vi "Demo.vi"() -> ()   [LabVIEW 2012]
panel:
  in  "MVOCX":refnum<k7>(container)
  out "采集BMP图像":picture
  in  "?":bool
  out "采集JPG图像":picture
  in  "Stop":bool
  in  "?":bool
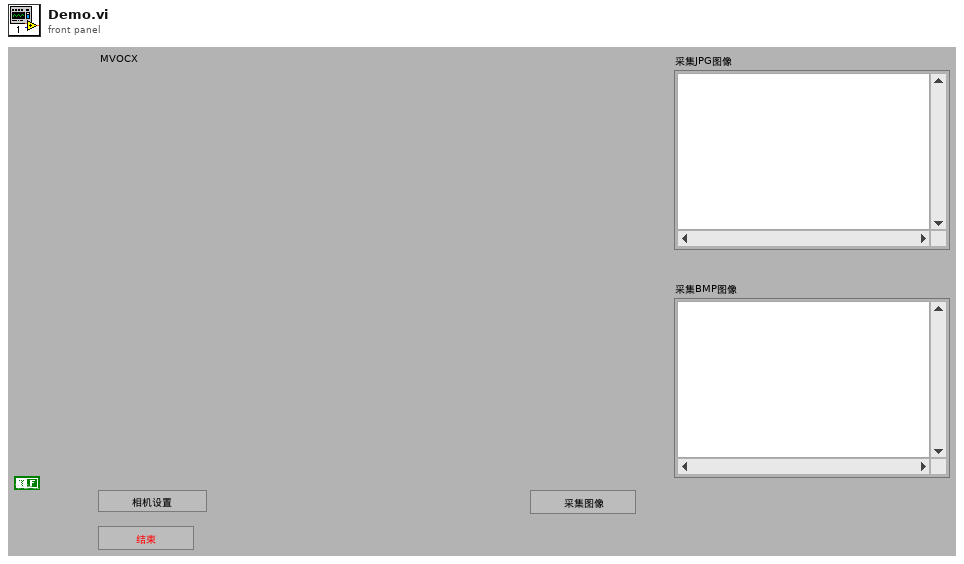
[diagram p1: front panel]
types:
  T1 = typedef "imagedata.ctl" = cluster{"image type":i32, "image depth":i32, "image":u8[], "mask":u8[], "colors":u32[], "Rectangle":cluster{"left":i16, "top":i16, "right":i16, "bottom":i16}}
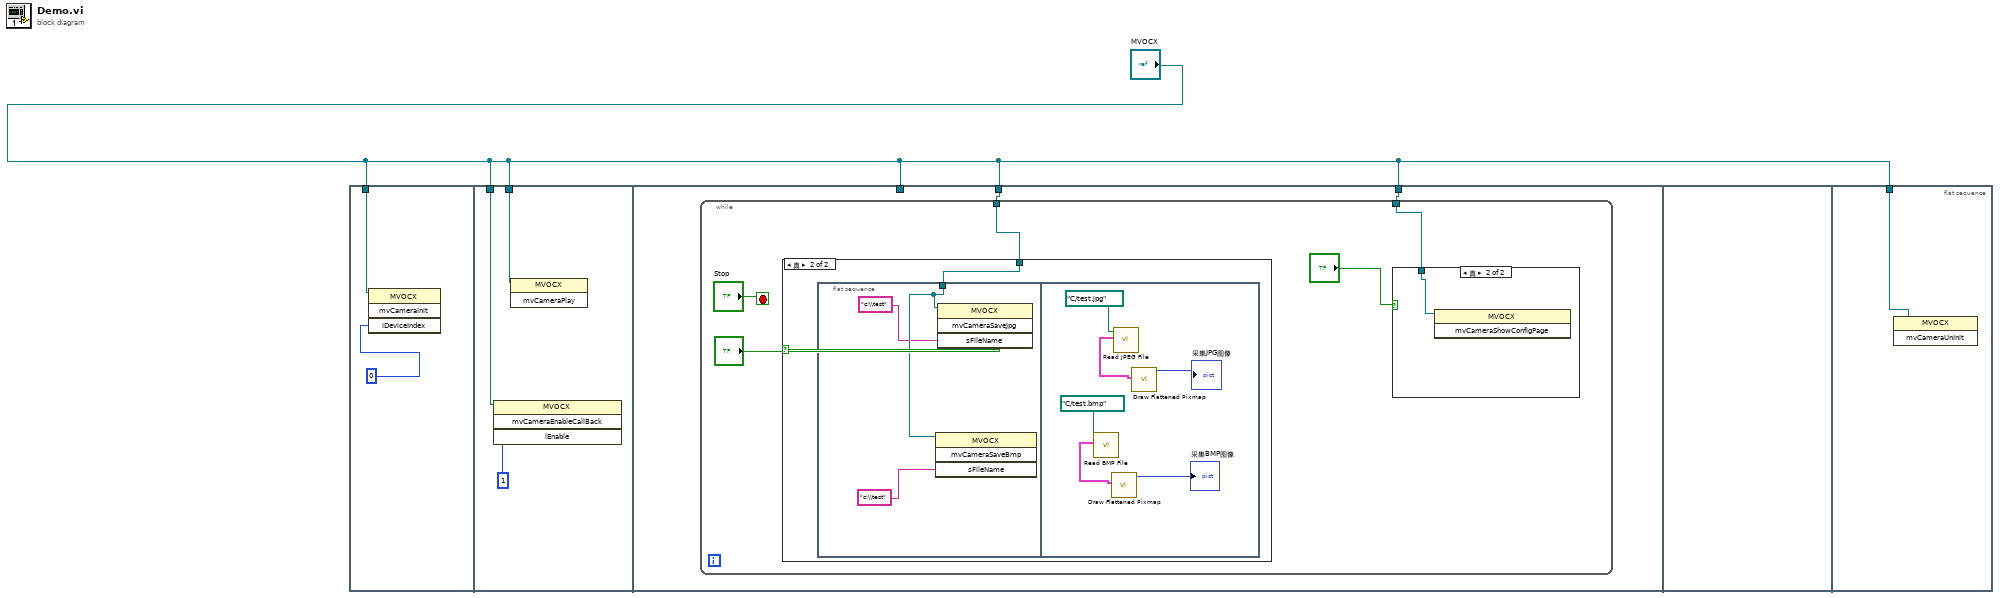
[diagram p0: block diagram]
diagram:
  n1 = flat-sequence {
    tunnel: "MVOCX" -> [w3]
    tunnel: "MVOCX" -> [w6]
    tunnel: "MVOCX" -> [w5]
    tunnel: "MVOCX" -> [_]
    tunnel: "MVOCX" -> [w8]
    tunnel: "MVOCX" -> [w7]
    tunnel: "MVOCX" -> [w25]
    frame #0 {
      n2 = invoke class="MVOCX" method="mvCameraInit"(reference=w3, "iDeviceIndex"=0) -> ()  [unwired: 2 in, 4 out]
    }
    frame #1 {
      n3 = invoke class="MVOCX" method="mvCameraEnableCallBack"(reference=w5, "lEnable"=1) -> ()  [unwired: 2 in, 4 out]
      n4 = invoke class="MVOCX" method="mvCameraPlay"(reference=w6) -> ()  [unwired: 2 in, 3 out]
    }
    frame #2 {
      n5 = while {
        tunnel: w8 -> [w9]
        tunnel: w7 -> [w10]
        stop <- "Stop" stop-if-true
        n6 = case shown="真" "?" {
          tunnel: w10 -> [_ w15]
          frame False {
          }
          frame True {
            n7 = flat-sequence {
              tunnel: w15 -> [w18]
              frame #0 {
                n8 = invoke class="MVOCX" method="mvCameraSaveBmp"(reference=w18, "sFileName"="c:\\test") -> ()  [unwired: 2 in, 4 out]
                n9 = invoke class="MVOCX" method="mvCameraSaveJpg"(reference=w18, "sFileName"="c:\\test") -> ()  [unwired: 2 in, 4 out]
              }
              frame #1 {
                n10 = call <vilib>:"Read BMP File.vi"("path to BMP file"=path "C:/test.bmp") -> ("image data"=w20:T1)  [unwired: 8 in, 2 out]
                n11 = call <vilib>:"Draw Flattened Pixmap.vi"("image data"=w20) -> ("new picture"=→"采集BMP图像":picture)  [unwired: 8 in]
                n12 = call <vilib>:"Read JPEG File.vi"("path to JPEG file"=path "C:/test.jpg" ("path to BMP file")) -> ("image data"=w23:T1)  [unwired: 8 in, 2 out]
                n13 = call <vilib>:"Draw Flattened Pixmap.vi"("image data"=w23) -> ("new picture"=→"采集JPG图像":picture)  [unwired: 8 in]
              }
            }
          }
        }
        n14 = case shown="真" "?" {
          tunnel: w9 -> [_ w14]
          frame False {
          }
          frame True {
            n15 = invoke class="MVOCX" method="mvCameraShowConfigPage"(reference=w14) -> ()  [unwired: 2 in, 3 out]
          }
        }
      }
    }
    frame #3 {
    }
    frame #4 {
      n16 = invoke class="MVOCX" method="mvCameraUnInit"(reference=w25) -> ()  [unwired: 2 in, 3 out]
    }
  }
